vi "S4GUI_003.vi"(7 "Tab ObsEng":enum32{"Obs", "CCD modes", "Guider", "Eng"}(tab)) -> ()   [LabVIEW 2018] (continued)
            n4197 = call "Write WPROT.vi"("error in (no error)"=w9692, "Opt_Selector.lvclass"=w9693, "Instrument in"=w9713) -> ("error out"=w9709:errorcluster, "Instrument out"=w9708:refnum<class "Instrument.lvclass">)  [unwired: 7 in]
            n4198 = call "Write Instrument.lvclass.vi"("error in (no error)"=w9709, "Instrument.lvclass"=w9708, "S4ACS_GUI in"=w9715) -> ("error out"=w9703:errorcluster, "S4ACS_GUI out"=w9691:refnum<class "S4GUI.lvclass">)  [unwired: 7 in]
          }
          frame Enabled {
            w9742 = FALSE ("Wait Until Done")
            n4199 = call <vilib>:"Application Directory.vi"() -> ("Application Directory"=w9737:path)
            n4200 = Build Path(base path=w9737, name or relative path="MsgAbort2.vi") -> (appended path=w9745:path)
            n4201 = Open VI Reference(vi path=w9745, error in (no error)=w9740) -> (vi reference=w9744:refnum<vi>, error out=w9743:errorcluster)  [unwired: 4 in]
            n4202 = invoke class="VI" method="Run VI"(reference=w9744, error in=w9743, "Wait until done"=w9742, "Auto Dispose Ref"=w9742) -> (error out=w9738:errorcluster)  [unwired: 1 in, 4 out]
          }
        }
      }
      event "Abort ch3": Value Change {
        n4203 = event-data() -> ()  [unwired: 1 in, 6 out]
        n4204 = disable-structure shown="Enabled" {
          disable-tunnel: w9749 -> [w9782 w9798]
          disable-tunnel: w9748 -> [w9780 w9799]
          disable-tunnel: [w9762 w9797] -> w9747
          disable-tunnel: [w9750 w9798] -> w9746
          frame Disabled {
            # "Para movimento \nda lamina retardadora"
            # "Restaura a última sequência de lâminas"
            n4205 = call-dynamic "Read AcquisitionC.vi"("error in (no error)"=w9780, "S4ACS_GUI in"=w9782) -> ("error out"=w9785:errorcluster, "Acquisition.lvclass"=w9784:refnum<class "Acquisition.lvclass">, "S4ACS_GUI out"=w9781:refnum<class "S4GUI.lvclass">)  [unwired: 7 in]
            n4206 = call-dynamic "Read Channel.vi"("error in (no error)"=w9785, "Acquisition in"=w9784) -> ("error out"=w9787:errorcluster, "Channel.lvclass"=w9786:refnum<class "Channel.lvclass">, "Acquisition out"=w9793:refnum<class "Acquisition.lvclass">)  [unwired: 7 in]
            n4207 = call-dynamic "Read State Machine.vi"("error in (no error)"=w9787, "Device in"=w9786) -> ("error out"=w9789:errorcluster, "State Machine.lvclass"=w9788:refnum<class "State Machine.lvclass">, "Device out"=w9791:refnum<class "Channel.lvclass">)  [unwired: 7 in]
            n4208 = call "Next State.vi"("error in (no error)"=w9789, "New_State"=u32 80, "State Machine in"=w9788) -> ("error out"=w9792:errorcluster, "State Machine out"=w9790:refnum<class "State Machine.lvclass">)  [unwired: 7 in]
            n4209 = call-dynamic "Write State Machine.vi"("error in (no error)"=w9792, "State Machine.lvclass"=w9790, "Device in"=w9791) -> ("error out"=w9794:errorcluster, "Device out"=w9795:refnum<class "Channel.lvclass">)  [unwired: 7 in]
            n4210 = call-dynamic "Write Channel.vi"("error in (no error)"=w9794, "Channel.lvclass"=w9795, "Acquisition in"=w9793) -> ("error out"=w9777:errorcluster, "Acquisition out"=w9778:refnum<class "Acquisition.lvclass">)  [unwired: 7 in]
            n4211 = call-dynamic "Write Acq_state.vi"("error in (no error)"=w9777, "Acq_state"=u32 0, "Acquisition in"=w9778) -> ("error out"=w9776:errorcluster, "Acquisition out"=w9775:refnum<class "Acquisition.lvclass">)  [unwired: 7 in]
            n4212 = call-dynamic "Write AcquisitionC.vi"("error in (no error)"=w9776, "Acquisition.lvclass"=w9775, "S4ACS_GUI in"=w9781) -> ("error out"=w9763:errorcluster, "S4ACS_GUI out"=w9761:refnum<class "S4GUI.lvclass">)  [unwired: 7 in]
            n4213 = call "Read Instrument.lvclass.vi"("error in (no error)"=w9763, "S4ACS_GUI in"=w9761) -> ("error out"=w9770:errorcluster, "Instrument.lvclass"=w9773:refnum<class "Instrument.lvclass">, "S4ACS_GUI out"=w9774:refnum<class "S4GUI.lvclass">)  [unwired: 7 in]
            n4214 = call "Read WPROT.vi"("error in (no error)"=w9770, "Instrument in"=w9773) -> ("error out"=w9769:errorcluster, "Opt_Selector.lvclass"=w9771:refnum<class "Opt_Selector.lvclass">, "Instrument out"=w9772:refnum<class "Instrument.lvclass">)  [unwired: 7 in]
            n4215 = call-dynamic "Read sequencia_ant.vi"("error in (no error)"=w9769, "Opt_Selector in"=w9771) -> ("error out"=w9765:errorcluster, "sequencia_ant"=w9764:u16, "Opt_Selector out"=w9766:refnum<class "Opt_Selector.lvclass">)  [unwired: 7 in]
            n4216 = call-dynamic "Write sequencia.vi"("error in (no error)"=w9765, "sequencia"=w9764, "Opt_Selector in"=w9766) -> ("error out"=w9754:errorcluster, "Opt_Selector out"=w9755:refnum<class "Opt_Selector.lvclass">)  [unwired: 7 in]
            n4217 = call-dynamic "Read State Machine.vi"("error in (no error)"=w9754, "Device in"=w9755) -> ("error out"=w9757:errorcluster, "State Machine.lvclass"=w9760:refnum<class "State Machine.lvclass">, "Device out"=w9753:refnum<class "Opt_Selector.lvclass">)  [unwired: 7 in]
            n4218 = call "Next State.vi"("error in (no error)"=w9757, "New_State"=10, "State Machine in"=w9760) -> ("error out"=w9756:errorcluster, "State Machine out"=w9759:refnum<class "State Machine.lvclass">)  [unwired: 7 in]
            n4219 = call-dynamic "Write State Machine.vi"("error in (no error)"=w9756, "State Machine.lvclass"=w9759, "Device in"=w9753) -> ("error out"=w9751:errorcluster, "Device out"=w9752:refnum<class "Opt_Selector.lvclass">)  [unwired: 7 in]
            n4220 = call "Write WPROT.vi"("error in (no error)"=w9751, "Opt_Selector.lvclass"=w9752, "Instrument in"=w9772) -> ("error out"=w9768:errorcluster, "Instrument out"=w9767:refnum<class "Instrument.lvclass">)  [unwired: 7 in]
            n4221 = call "Write Instrument.lvclass.vi"("error in (no error)"=w9768, "Instrument.lvclass"=w9767, "S4ACS_GUI in"=w9774) -> ("error out"=w9762:errorcluster, "S4ACS_GUI out"=w9750:refnum<class "S4GUI.lvclass">)  [unwired: 7 in]
          }
          frame Enabled {
            w9801 = FALSE ("Wait Until Done")
            n4222 = call <vilib>:"Application Directory.vi"() -> ("Application Directory"=w9796:path)
            n4223 = Build Path(base path=w9796, name or relative path="MsgAbort3.vi") -> (appended path=w9804:path)
            n4224 = Open VI Reference(vi path=w9804, error in (no error)=w9799) -> (vi reference=w9803:refnum<vi>, error out=w9802:errorcluster)  [unwired: 4 in]
            n4225 = invoke class="VI" method="Run VI"(reference=w9803, error in=w9802, "Wait until done"=w9801, "Auto Dispose Ref"=w9801) -> (error out=w9797:errorcluster)  [unwired: 1 in, 4 out]
          }
        }
      }
      event "Abort ch4": Value Change {
        n4226 = event-data() -> ()  [unwired: 1 in, 6 out]
        n4227 = disable-structure shown="Enabled" {
          disable-tunnel: w9808 -> [w9841 w9857]
          disable-tunnel: w9807 -> [w9839 w9858]
          disable-tunnel: [w9821 w9856] -> w9806
          disable-tunnel: [w9809 w9857] -> w9805
          frame Disabled {
            # "Para movimento \nda lamina retardadora"
            # "Restaura a última sequência de lâminas"
            n4228 = call-dynamic "Read AcquisitionD.vi"("error in (no error)"=w9839, "S4ACS_GUI in"=w9841) -> ("error out"=w9844:errorcluster, "Acquisition.lvclass"=w9843:refnum<class "Acquisition.lvclass">, "S4ACS_GUI out"=w9840:refnum<class "S4GUI.lvclass">)  [unwired: 7 in]
            n4229 = call-dynamic "Read Channel.vi"("error in (no error)"=w9844, "Acquisition in"=w9843) -> ("error out"=w9846:errorcluster, "Channel.lvclass"=w9845:refnum<class "Channel.lvclass">, "Acquisition out"=w9852:refnum<class "Acquisition.lvclass">)  [unwired: 7 in]
            n4230 = call-dynamic "Read State Machine.vi"("error in (no error)"=w9846, "Device in"=w9845) -> ("error out"=w9848:errorcluster, "State Machine.lvclass"=w9847:refnum<class "State Machine.lvclass">, "Device out"=w9850:refnum<class "Channel.lvclass">)  [unwired: 7 in]
            n4231 = call "Next State.vi"("error in (no error)"=w9848, "New_State"=u32 80, "State Machine in"=w9847) -> ("error out"=w9851:errorcluster, "State Machine out"=w9849:refnum<class "State Machine.lvclass">)  [unwired: 7 in]
            n4232 = call-dynamic "Write State Machine.vi"("error in (no error)"=w9851, "State Machine.lvclass"=w9849, "Device in"=w9850) -> ("error out"=w9853:errorcluster, "Device out"=w9854:refnum<class "Channel.lvclass">)  [unwired: 7 in]
            n4233 = call-dynamic "Write Channel.vi"("error in (no error)"=w9853, "Channel.lvclass"=w9854, "Acquisition in"=w9852) -> ("error out"=w9836:errorcluster, "Acquisition out"=w9837:refnum<class "Acquisition.lvclass">)  [unwired: 7 in]
            n4234 = call-dynamic "Write Acq_state.vi"("error in (no error)"=w9836, "Acq_state"=u32 0, "Acquisition in"=w9837) -> ("error out"=w9835:errorcluster, "Acquisition out"=w9834:refnum<class "Acquisition.lvclass">)  [unwired: 7 in]
            n4235 = call-dynamic "Write AcquisitionD.vi"("error in (no error)"=w9835, "Acquisition.lvclass"=w9834, "S4ACS_GUI in"=w9840) -> ("error out"=w9822:errorcluster, "S4ACS_GUI out"=w9820:refnum<class "S4GUI.lvclass">)  [unwired: 7 in]
            n4236 = call "Read Instrument.lvclass.vi"("error in (no error)"=w9822, "S4ACS_GUI in"=w9820) -> ("error out"=w9829:errorcluster, "Instrument.lvclass"=w9832:refnum<class "Instrument.lvclass">, "S4ACS_GUI out"=w9833:refnum<class "S4GUI.lvclass">)  [unwired: 7 in]
            n4237 = call "Read WPROT.vi"("error in (no error)"=w9829, "Instrument in"=w9832) -> ("error out"=w9828:errorcluster, "Opt_Selector.lvclass"=w9830:refnum<class "Opt_Selector.lvclass">, "Instrument out"=w9831:refnum<class "Instrument.lvclass">)  [unwired: 7 in]
            n4238 = call-dynamic "Read sequencia_ant.vi"("error in (no error)"=w9828, "Opt_Selector in"=w9830) -> ("error out"=w9824:errorcluster, "sequencia_ant"=w9823:u16, "Opt_Selector out"=w9825:refnum<class "Opt_Selector.lvclass">)  [unwired: 7 in]
            n4239 = call-dynamic "Write sequencia.vi"("error in (no error)"=w9824, "sequencia"=w9823, "Opt_Selector in"=w9825) -> ("error out"=w9813:errorcluster, "Opt_Selector out"=w9814:refnum<class "Opt_Selector.lvclass">)  [unwired: 7 in]
            n4240 = call-dynamic "Read State Machine.vi"("error in (no error)"=w9813, "Device in"=w9814) -> ("error out"=w9816:errorcluster, "State Machine.lvclass"=w9819:refnum<class "State Machine.lvclass">, "Device out"=w9812:refnum<class "Opt_Selector.lvclass">)  [unwired: 7 in]
            n4241 = call "Next State.vi"("error in (no error)"=w9816, "New_State"=10, "State Machine in"=w9819) -> ("error out"=w9815:errorcluster, "State Machine out"=w9818:refnum<class "State Machine.lvclass">)  [unwired: 7 in]
            n4242 = call-dynamic "Write State Machine.vi"("error in (no error)"=w9815, "State Machine.lvclass"=w9818, "Device in"=w9812) -> ("error out"=w9810:errorcluster, "Device out"=w9811:refnum<class "Opt_Selector.lvclass">)  [unwired: 7 in]
            n4243 = call "Write WPROT.vi"("error in (no error)"=w9810, "Opt_Selector.lvclass"=w9811, "Instrument in"=w9831) -> ("error out"=w9827:errorcluster, "Instrument out"=w9826:refnum<class "Instrument.lvclass">)  [unwired: 7 in]
            n4244 = call "Write Instrument.lvclass.vi"("error in (no error)"=w9827, "Instrument.lvclass"=w9826, "S4ACS_GUI in"=w9833) -> ("error out"=w9821:errorcluster, "S4ACS_GUI out"=w9809:refnum<class "S4GUI.lvclass">)  [unwired: 7 in]
          }
          frame Enabled {
            w9860 = FALSE ("Wait Until Done")
            n4245 = call <vilib>:"Application Directory.vi"() -> ("Application Directory"=w9855:path)
            n4246 = Build Path(base path=w9855, name or relative path="MsgAbort4.vi") -> (appended path=w9863:path)
            n4247 = Open VI Reference(vi path=w9863, error in (no error)=w9858) -> (vi reference=w9862:refnum<vi>, error out=w9861:errorcluster)  [unwired: 4 in]
            n4248 = invoke class="VI" method="Run VI"(reference=w9862, error in=w9861, "Wait until done"=w9860, "Auto Dispose Ref"=w9860) -> (error out=w9856:errorcluster)  [unwired: 1 in, 4 out]
          }
        }
      }
      event "SyncBox": Value Change {
        n4249 = event-data() -> ()  [unwired: 1 in, 4 out]
        n4250 = call-dynamic "Read Sync Box.lvclass.vi"("error in (no error)"=w9866, "SPARC4_AC in"=w9867) -> ("error out"=w9882:errorcluster, "Sync Box.lvclass"=w9883:refnum<class "Sync Box.lvclass">, "SPARC4_AC out"=w9871:refnum<class "S4GUI.lvclass">)  [unwired: 7 in]
        n4251 = call-dynamic "Read Trigger.lvclass.vi"("error in (no error)"=w9882, "Sync Box in"=w9883) -> ("error out"=w9880:errorcluster, "Trigger.lvclass"=w9881:refnum<class "Trigger.lvclass">, "Sync Box out"=w9874:refnum<class "Sync Box.lvclass">)  [unwired: 7 in]
        n4252 = call-dynamic "Read State Machine.vi"("error in (no error)"=w9880, "Device in"=w9881) -> ("error out"=w9878:errorcluster, "State Machine.lvclass"=w9879:refnum<class "State Machine.lvclass">, "Device out"=w9875:refnum<class "Trigger.lvclass">)  [unwired: 7 in]
        n4253 = call "Next State.vi"("error in (no error)"=w9878, "New_State"=u32 1, "State Machine in"=w9879) -> ("error out"=w9873:errorcluster, "State Machine out"=w9876:refnum<class "State Machine.lvclass">)  [unwired: 7 in]
        n4254 = call-dynamic "Write State Machine.vi"("error in (no error)"=w9873, "State Machine.lvclass"=w9876, "Device in"=w9875) -> ("error out"=w9869:errorcluster, "Device out"=w9868:refnum<class "Trigger.lvclass">)  [unwired: 7 in]
        n4255 = call-dynamic "Write Trigger.lvclass.vi"("error in (no error)"=w9869, "Trigger.lvclass"=w9868, "Sync Box in"=w9874) -> ("error out"=w9870:errorcluster, "Sync Box out"=w9872:refnum<class "Sync Box.lvclass">)  [unwired: 7 in]
        n4256 = call-dynamic "Write Sync Box.lvclass.vi"("error in (no error)"=w9870, "Sync Box.lvclass"=w9872, "SPARC4_AC in"=w9871) -> ("error out"=w9865:errorcluster, "SPARC4_AC out"=w9864:refnum<class "S4GUI.lvclass">)  [unwired: 7 in]
      }
      event "Fire manual", "Fire": Value Change {
        n4257 = event-data() -> ()  [unwired: 1 in, 4 out]
        n4258 = call-dynamic "Read Sync Box.lvclass.vi"("error in (no error)"=w9886, "SPARC4_AC in"=w9887) -> ("error out"=w9902:errorcluster, "Sync Box.lvclass"=w9903:refnum<class "Sync Box.lvclass">, "SPARC4_AC out"=w9891:refnum<class "S4GUI.lvclass">)  [unwired: 7 in]
        n4259 = call-dynamic "Read Trigger.lvclass.vi"("error in (no error)"=w9902, "Sync Box in"=w9903) -> ("error out"=w9900:errorcluster, "Trigger.lvclass"=w9901:refnum<class "Trigger.lvclass">, "Sync Box out"=w9894:refnum<class "Sync Box.lvclass">)  [unwired: 7 in]
        n4260 = call-dynamic "Read State Machine.vi"("error in (no error)"=w9900, "Device in"=w9901) -> ("error out"=w9898:errorcluster, "State Machine.lvclass"=w9899:refnum<class "State Machine.lvclass">, "Device out"=w9895:refnum<class "Trigger.lvclass">)  [unwired: 7 in]
        n4261 = call "Next State.vi"("error in (no error)"=w9898, "New_State"=u32 40, "State Machine in"=w9899) -> ("error out"=w9893:errorcluster, "State Machine out"=w9896:refnum<class "State Machine.lvclass">)  [unwired: 7 in]
        n4262 = call-dynamic "Write State Machine.vi"("error in (no error)"=w9893, "State Machine.lvclass"=w9896, "Device in"=w9895) -> ("error out"=w9889:errorcluster, "Device out"=w9888:refnum<class "Trigger.lvclass">)  [unwired: 7 in]
        n4263 = call-dynamic "Write Trigger.lvclass.vi"("error in (no error)"=w9889, "Trigger.lvclass"=w9888, "Sync Box in"=w9894) -> ("error out"=w9890:errorcluster, "Sync Box out"=w9892:refnum<class "Sync Box.lvclass">)  [unwired: 7 in]
        n4264 = call-dynamic "Write Sync Box.lvclass.vi"("error in (no error)"=w9890, "Sync Box.lvclass"=w9892, "SPARC4_AC in"=w9891) -> ("error out"=w9885:errorcluster, "SPARC4_AC out"=w9884:refnum<class "S4GUI.lvclass">)  [unwired: 7 in]
      }
      event "Select Trigger Mode": Value Change {
        n4265 = event-data() -> ("NewVal"=w9905:bool)  [unwired: 1 in, 2 out]
        n4266 = call-dynamic "Read Sync Box.lvclass.vi"("error in (no error)"=w9913, "SPARC4_AC in"=w9914) -> ("error out"=w9925:errorcluster, "Sync Box.lvclass"=w9926:refnum<class "Sync Box.lvclass">, "SPARC4_AC out"=w9918:refnum<class "S4GUI.lvclass">)  [unwired: 7 in]
        n4267 = call-dynamic "Read Trigger.lvclass.vi"("error in (no error)"=w9925, "Sync Box in"=w9926) -> ("error out"=w9906:errorcluster, "Trigger.lvclass"=w9909:refnum<class "Trigger.lvclass">, "Sync Box out"=w9921:refnum<class "Sync Box.lvclass">)  [unwired: 7 in]
        n4268 = call-dynamic "Write Trigger Mode Target.vi"("error in (no error)"=w9906, "Trigger Mode Target"=w9905, "Trigger in"=w9909) -> ("error out"=w9907:errorcluster, "Trigger out"=w9908:refnum<class "Trigger.lvclass">)  [unwired: 7 in]
        n4269 = call-dynamic "Read State Machine.vi"("error in (no error)"=w9907, "Device in"=w9908) -> ("error out"=w9910:errorcluster, "State Machine.lvclass"=w9911:refnum<class "State Machine.lvclass">, "Device out"=w9922:refnum<class "Trigger.lvclass">)  [unwired: 7 in]
        n4270 = call "Next State.vi"("error in (no error)"=w9910, "New_State"=u32 30, "State Machine in"=w9911) -> ("error out"=w9920:errorcluster, "State Machine out"=w9923:refnum<class "State Machine.lvclass">)  [unwired: 7 in]
        n4271 = call-dynamic "Write State Machine.vi"("error in (no error)"=w9920, "State Machine.lvclass"=w9923, "Device in"=w9922) -> ("error out"=w9916:errorcluster, "Device out"=w9915:refnum<class "Trigger.lvclass">)  [unwired: 7 in]
        n4272 = call-dynamic "Write Trigger.lvclass.vi"("error in (no error)"=w9916, "Trigger.lvclass"=w9915, "Sync Box in"=w9921) -> ("error out"=w9917:errorcluster, "Sync Box out"=w9919:refnum<class "Sync Box.lvclass">)  [unwired: 7 in]
        n4273 = call-dynamic "Write Sync Box.lvclass.vi"("error in (no error)"=w9917, "Sync Box.lvclass"=w9919, "SPARC4_AC in"=w9918) -> ("error out"=w9912:errorcluster, "SPARC4_AC out"=w9904:refnum<class "S4GUI.lvclass">)  [unwired: 7 in]
      }
      event "Set SyncBox": Value Change {
        n4274 = event-data() -> ()  [unwired: 1 in, 4 out]
        n4275 = call-dynamic "Read Sync Box.lvclass.vi"("error in (no error)"=w9929, "SPARC4_AC in"=w9930) -> ("error out"=w9945:errorcluster, "Sync Box.lvclass"=w9946:refnum<class "Sync Box.lvclass">, "SPARC4_AC out"=w9934:refnum<class "S4GUI.lvclass">)  [unwired: 7 in]
        n4276 = call-dynamic "Read Trigger.lvclass.vi"("error in (no error)"=w9945, "Sync Box in"=w9946) -> ("error out"=w9943:errorcluster, "Trigger.lvclass"=w9944:refnum<class "Trigger.lvclass">, "Sync Box out"=w9937:refnum<class "Sync Box.lvclass">)  [unwired: 7 in]
        n4277 = call-dynamic "Read State Machine.vi"("error in (no error)"=w9943, "Device in"=w9944) -> ("error out"=w9941:errorcluster, "State Machine.lvclass"=w9942:refnum<class "State Machine.lvclass">, "Device out"=w9938:refnum<class "Trigger.lvclass">)  [unwired: 7 in]
        n4278 = call "Next State.vi"("error in (no error)"=w9941, "New_State"=u32 10, "State Machine in"=w9942) -> ("error out"=w9936:errorcluster, "State Machine out"=w9939:refnum<class "State Machine.lvclass">)  [unwired: 7 in]
        n4279 = call-dynamic "Write State Machine.vi"("error in (no error)"=w9936, "State Machine.lvclass"=w9939, "Device in"=w9938) -> ("error out"=w9932:errorcluster, "Device out"=w9931:refnum<class "Trigger.lvclass">)  [unwired: 7 in]
        n4280 = call-dynamic "Write Trigger.lvclass.vi"("error in (no error)"=w9932, "Trigger.lvclass"=w9931, "Sync Box in"=w9937) -> ("error out"=w9933:errorcluster, "Sync Box out"=w9935:refnum<class "Sync Box.lvclass">)  [unwired: 7 in]
        n4281 = call-dynamic "Write Sync Box.lvclass.vi"("error in (no error)"=w9933, "Sync Box.lvclass"=w9935, "SPARC4_AC in"=w9934) -> ("error out"=w9928:errorcluster, "SPARC4_AC out"=w9927:refnum<class "S4GUI.lvclass">)  [unwired: 7 in]
      }
      event "Set Focus": Value Change {
        n4282 = event-data() -> ("NewVal"=w9947:bool)  [unwired: 1 in]
        n4283 = case shown="True" w9947 {
          tunnel: w9951 -> [w9953 w9962]
          tunnel: w9950 -> [w9952 w9961]
          tunnel: [w9952 w9960] -> w9949
          tunnel: [w9953 w9959] -> w9948
          frame False {
          }
          frame True {
            n4284 = call-dynamic "Read TelFocus.lvclass.vi"("error in (no error)"=w9961, "S4GUI in"=w9962) -> ("error out"=w9975:errorcluster, "TelFocus.lvclass"=w9976:refnum<class "TelFocus.lvclass">, "S4GUI out"=w9966:refnum<class "S4GUI.lvclass">)  [unwired: 7 in]
            n4285 = call-dynamic "Read SecMirror.lvclass.vi"("error in (no error)"=w9975, "TelFocus in"=w9976) -> ("error out"=w9955:errorcluster, "SecMirror.lvclass"=w9958:refnum<class "SecMirror.lvclass">, "TelFocus out"=w9969:refnum<class "TelFocus.lvclass">)  [unwired: 7 in]
            n4286 = call-dynamic "Write target.vi"("error in (no error)"=w9955, "target"="Target focus", "SecMirror in"=w9958) -> ("error out"=w9954:errorcluster, "SecMirror out"=w9957:refnum<class "SecMirror.lvclass">)  [unwired: 7 in]
            n4287 = call-dynamic "Read State Machine.vi"("error in (no error)"=w9954, "Device in"=w9957) -> ("error out"=w9973:errorcluster, "State Machine.lvclass"=w9974:refnum<class "State Machine.lvclass">, "Device out"=w9970:refnum<class "SecMirror.lvclass">)  [unwired: 7 in]
            n4288 = call "Next State.vi"("error in (no error)"=w9973, "New_State"=1, "State Machine in"=w9974) -> ("error out"=w9968:errorcluster, "State Machine out"=w9971:refnum<class "State Machine.lvclass">)  [unwired: 7 in]
            n4289 = call-dynamic "Write State Machine.vi"("error in (no error)"=w9968, "State Machine.lvclass"=w9971, "Device in"=w9970) -> ("error out"=w9964:errorcluster, "Device out"=w9963:refnum<class "SecMirror.lvclass">)  [unwired: 7 in]
            n4290 = call-dynamic "Write SecMirror.lvclass.vi"("error in (no error)"=w9964, "SecMirror.lvclass"=w9963, "TelFocus in"=w9969) -> ("error out"=w9965:errorcluster, "TelFocus out"=w9967:refnum<class "TelFocus.lvclass">)  [unwired: 7 in]
            n4291 = call-dynamic "Write TelFocus.lvclass.vi"("error in (no error)"=w9965, "TelFocus.lvclass"=w9967, "S4GUI in"=w9966) -> ("error out"=w9960:errorcluster, "S4GUI out"=w9959:refnum<class "S4GUI.lvclass">)  [unwired: 7 in]
          }
        }
      }
      event "Set Focus 2": Value Change {
        n4292 = event-data() -> ("NewVal"=w9977:bool)  [unwired: 1 in]
        n4293 = case shown="True" w9977 {
          tunnel: w9981 -> [w9983 w9992]
          tunnel: w9980 -> [w9982 w9991]
          tunnel: [w9982 w9990] -> w9979
          tunnel: [w9983 w9989] -> w9978
          frame False {
          }
          frame True {
            n4294 = call-dynamic "Read TelFocus.lvclass.vi"("error in (no error)"=w9991, "S4GUI in"=w9992) -> ("error out"=w10005:errorcluster, "TelFocus.lvclass"=w10006:refnum<class "TelFocus.lvclass">, "S4GUI out"=w9996:refnum<class "S4GUI.lvclass">)  [unwired: 7 in]
            n4295 = call-dynamic "Read SecMirror.lvclass.vi"("error in (no error)"=w10005, "TelFocus in"=w10006) -> ("error out"=w9986:errorcluster, "SecMirror.lvclass"=w9988:refnum<class "SecMirror.lvclass">, "TelFocus out"=w9999:refnum<class "TelFocus.lvclass">)  [unwired: 7 in]
            n4296 = call-dynamic "Write target.vi"("error in (no error)"=w9986, "target"="Target focus 2", "SecMirror in"=w9988) -> ("error out"=w9985:errorcluster, "SecMirror out"=w9987:refnum<class "SecMirror.lvclass">)  [unwired: 7 in]
            n4297 = call-dynamic "Read State Machine.vi"("error in (no error)"=w9985, "Device in"=w9987) -> ("error out"=w10003:errorcluster, "State Machine.lvclass"=w10004:refnum<class "State Machine.lvclass">, "Device out"=w10000:refnum<class "SecMirror.lvclass">)  [unwired: 7 in]
            n4298 = call "Next State.vi"("error in (no error)"=w10003, "New_State"=1, "State Machine in"=w10004) -> ("error out"=w9998:errorcluster, "State Machine out"=w10001:refnum<class "State Machine.lvclass">)  [unwired: 7 in]
            n4299 = call-dynamic "Write State Machine.vi"("error in (no error)"=w9998, "State Machine.lvclass"=w10001, "Device in"=w10000) -> ("error out"=w9994:errorcluster, "Device out"=w9993:refnum<class "SecMirror.lvclass">)  [unwired: 7 in]
            n4300 = call-dynamic "Write SecMirror.lvclass.vi"("error in (no error)"=w9994, "SecMirror.lvclass"=w9993, "TelFocus in"=w9999) -> ("error out"=w9995:errorcluster, "TelFocus out"=w9997:refnum<class "TelFocus.lvclass">)  [unwired: 7 in]
            n4301 = call-dynamic "Write TelFocus.lvclass.vi"("error in (no error)"=w9995, "TelFocus.lvclass"=w9997, "S4GUI in"=w9996) -> ("error out"=w9990:errorcluster, "S4GUI out"=w9989:refnum<class "S4GUI.lvclass">)  [unwired: 7 in]
          }
        }
      }
      event "Stop Focus", "Stop Focus 2": Value Change {
        n4302 = event-data() -> ("NewVal"=w10007:bool)  [unwired: 1 in]
        n4303 = case shown="True" w10007 {
          tunnel: w10011 -> [w10013 w10019]
          tunnel: w10010 -> [w10012 w10018]
          tunnel: [w10012 w10017] -> w10009
          tunnel: [w10013 w10016] -> w10008
          frame False {
          }
          frame True {
            n4304 = call-dynamic "Read TelFocus.lvclass.vi"("error in (no error)"=w10018, "S4GUI in"=w10019) -> ("error out"=w10032:errorcluster, "TelFocus.lvclass"=w10033:refnum<class "TelFocus.lvclass">, "S4GUI out"=w10023:refnum<class "S4GUI.lvclass">)  [unwired: 7 in]
            n4305 = call-dynamic "Read SecMirror.lvclass.vi"("error in (no error)"=w10032, "TelFocus in"=w10033) -> ("error out"=w10014:errorcluster, "SecMirror.lvclass"=w10015:refnum<class "SecMirror.lvclass">, "TelFocus out"=w10026:refnum<class "TelFocus.lvclass">)  [unwired: 7 in]
            n4306 = call-dynamic "Read State Machine.vi"("error in (no error)"=w10014, "Device in"=w10015) -> ("error out"=w10030:errorcluster, "State Machine.lvclass"=w10031:refnum<class "State Machine.lvclass">, "Device out"=w10027:refnum<class "SecMirror.lvclass">)  [unwired: 7 in]
            n4307 = call "Next State.vi"("error in (no error)"=w10030, "New_State"=10, "State Machine in"=w10031) -> ("error out"=w10025:errorcluster, "State Machine out"=w10028:refnum<class "State Machine.lvclass">)  [unwired: 7 in]
            n4308 = call-dynamic "Write State Machine.vi"("error in (no error)"=w10025, "State Machine.lvclass"=w10028, "Device in"=w10027) -> ("error out"=w10021:errorcluster, "Device out"=w10020:refnum<class "SecMirror.lvclass">)  [unwired: 7 in]
            n4309 = call-dynamic "Write SecMirror.lvclass.vi"("error in (no error)"=w10021, "SecMirror.lvclass"=w10020, "TelFocus in"=w10026) -> ("error out"=w10022:errorcluster, "TelFocus out"=w10024:refnum<class "TelFocus.lvclass">)  [unwired: 7 in]
            n4310 = call-dynamic "Write TelFocus.lvclass.vi"("error in (no error)"=w10022, "TelFocus.lvclass"=w10024, "S4GUI in"=w10023) -> ("error out"=w10017:errorcluster, "S4GUI out"=w10016:refnum<class "S4GUI.lvclass">)  [unwired: 7 in]
          }
        }
      }
      event "cooler ON 1": Value Change {
        n4311 = event-data() -> ("NewVal"=w10034:bool)  [unwired: 1 in]
        n4312 = case shown="True" w10034 {
          tunnel: [w10039 w10074] -> w10038
          tunnel: [w10040 w10073] -> w10037
          tunnel: w10036 -> [w10040 w10044]
          tunnel: w10035 -> [w10039 w10043]
          frame False {
          }
          frame True {
            w10042 = i16 1 items=["Cooler OFF", "Cooler ON"] ("Cooler ON/OFF")
            n4313 = Concatenate Strings("SET COOLER " ("User Event"), "ON ", "CLICKED - CH1" ("User Event")) -> (w10046:string)
            n4314 = call-dynamic "Write User Event.vi"("error in (no error)"=w10043, "User Event"=w10046, "S4GUI in"=w10044) -> ("error out"=w10047:errorcluster, "S4GUI out"=w10049:refnum<class "S4GUI.lvclass">)  [unwired: 7 in]
            n4315 = call-dynamic "Read AcquisitionA.vi"("error in (no error)"=w10047, "S4ACS_GUI in"=w10049) -> ("error out"=w10071:errorcluster, "Acquisition.lvclass"=w10072:refnum<class "Acquisition.lvclass">, "S4ACS_GUI out"=w10062:refnum<class "S4GUI.lvclass">)  [unwired: 7 in]
            n4316 = call-dynamic "Read Channel.vi"("error in (no error)"=w10071, "Acquisition in"=w10072) -> ("error out"=w10055:errorcluster, "Channel.lvclass"=w10059:refnum<class "Channel.lvclass">, "Acquisition out"=w10065:refnum<class "Acquisition.lvclass">)  [unwired: 7 in]
            n4317 = call-dynamic "Read Interface.vi"("error in (no error)"=w10055, "Channel in"=w10059) -> ("error out"=w10050:errorcluster, "Interface.lvclass"=w10051:refnum<class "Interface.lvclass">, "Channel out"=w10058:refnum<class "Channel.lvclass">)  [unwired: 7 in]
            n4318 = call-dynamic "Write Cooler ON_OFF.vi"("error in (no error)"=w10050, "Cooler ON/OFF"=w10042, "Interface in"=w10051) -> ("error out"=w10054:errorcluster, "Interface out"=w10056:refnum<class "Interface.lvclass">)  [unwired: 7 in]
            n4319 = call-dynamic "Write Interface.vi"("error in (no error)"=w10054, "Interface.lvclass"=w10056, "Channel in"=w10058) -> ("error out"=w10053:errorcluster, "Channel out"=w10057:refnum<class "Channel.lvclass">)  [unwired: 7 in]
            n4320 = call-dynamic "Read State Machine.vi"("error in (no error)"=w10053, "Device in"=w10057) -> ("error out"=w10069:errorcluster, "State Machine.lvclass"=w10070:refnum<class "State Machine.lvclass">, "Device out"=w10066:refnum<class "Channel.lvclass">)  [unwired: 7 in]
            n4321 = call "Next State.vi"("error in (no error)"=w10069, "New_State"=u32 30, "State Machine in"=w10070) -> ("error out"=w10064:errorcluster, "State Machine out"=w10067:refnum<class "State Machine.lvclass">)  [unwired: 7 in]
            n4322 = call-dynamic "Write State Machine.vi"("error in (no error)"=w10064, "State Machine.lvclass"=w10067, "Device in"=w10066) -> ("error out"=w10060:errorcluster, "Device out"=w10052:refnum<class "Channel.lvclass">)  [unwired: 7 in]
            n4323 = call-dynamic "Write Channel.vi"("error in (no error)"=w10060, "Channel.lvclass"=w10052, "Acquisition in"=w10065) -> ("error out"=w10061:errorcluster, "Acquisition out"=w10063:refnum<class "Acquisition.lvclass">)  [unwired: 7 in]
            n4324 = call-dynamic "Write AcquisitionA.vi"("error in (no error)"=w10061, "Acquisition.lvclass"=w10063, "S4ACS_GUI in"=w10062) -> ("error out"=w10074:errorcluster, "S4ACS_GUI out"=w10073:refnum<class "S4GUI.lvclass">)  [unwired: 7 in]
          }
        }
      }
      event "cooler ON 2": Value Change {
        n4325 = event-data() -> ("NewVal"=w10075:bool)  [unwired: 1 in]
        n4326 = case shown="True" w10075 {
          tunnel: [w10080 w10115] -> w10079
          tunnel: [w10081 w10114] -> w10078
          tunnel: w10077 -> [w10081 w10085]
          tunnel: w10076 -> [w10080 w10084]
          frame False {
          }
          frame True {
            w10083 = i16 1 items=["Cooler OFF", "Cooler ON"] ("Cooler ON/OFF")
            n4327 = Concatenate Strings("SET COOLER " ("User Event"), "ON ", "CLICKED - CH2" ("User Event")) -> (w10087:string)
            n4328 = call-dynamic "Write User Event.vi"("error in (no error)"=w10084, "User Event"=w10087, "S4GUI in"=w10085) -> ("error out"=w10088:errorcluster, "S4GUI out"=w10090:refnum<class "S4GUI.lvclass">)  [unwired: 7 in]
            n4329 = call "Read AcquisitionB.vi"("error in (no error)"=w10088, "S4ACS_GUI in"=w10090) -> ("error out"=w10112:errorcluster, "Acquisition.lvclass"=w10113:refnum<class "Acquisition.lvclass">, "S4ACS_GUI out"=w10103:refnum<class "S4GUI.lvclass">)  [unwired: 7 in]
            n4330 = call-dynamic "Read Channel.vi"("error in (no error)"=w10112, "Acquisition in"=w10113) -> ("error out"=w10096:errorcluster, "Channel.lvclass"=w10100:refnum<class "Channel.lvclass">, "Acquisition out"=w10106:refnum<class "Acquisition.lvclass">)  [unwired: 7 in]
            n4331 = call-dynamic "Read Interface.vi"("error in (no error)"=w10096, "Channel in"=w10100) -> ("error out"=w10091:errorcluster, "Interface.lvclass"=w10092:refnum<class "Interface.lvclass">, "Channel out"=w10099:refnum<class "Channel.lvclass">)  [unwired: 7 in]
            n4332 = call-dynamic "Write Cooler ON_OFF.vi"("error in (no error)"=w10091, "Cooler ON/OFF"=w10083, "Interface in"=w10092) -> ("error out"=w10095:errorcluster, "Interface out"=w10097:refnum<class "Interface.lvclass">)  [unwired: 7 in]
            n4333 = call-dynamic "Write Interface.vi"("error in (no error)"=w10095, "Interface.lvclass"=w10097, "Channel in"=w10099) -> ("error out"=w10094:errorcluster, "Channel out"=w10098:refnum<class "Channel.lvclass">)  [unwired: 7 in]
            n4334 = call-dynamic "Read State Machine.vi"("error in (no error)"=w10094, "Device in"=w10098) -> ("error out"=w10110:errorcluster, "State Machine.lvclass"=w10111:refnum<class "State Machine.lvclass">, "Device out"=w10107:refnum<class "Channel.lvclass">)  [unwired: 7 in]
            n4335 = call "Next State.vi"("error in (no error)"=w10110, "New_State"=u32 30, "State Machine in"=w10111) -> ("error out"=w10105:errorcluster, "State Machine out"=w10108:refnum<class "State Machine.lvclass">)  [unwired: 7 in]
            n4336 = call-dynamic "Write State Machine.vi"("error in (no error)"=w10105, "State Machine.lvclass"=w10108, "Device in"=w10107) -> ("error out"=w10101:errorcluster, "Device out"=w10093:refnum<class "Channel.lvclass">)  [unwired: 7 in]
            n4337 = call-dynamic "Write Channel.vi"("error in (no error)"=w10101, "Channel.lvclass"=w10093, "Acquisition in"=w10106) -> ("error out"=w10102:errorcluster, "Acquisition out"=w10104:refnum<class "Acquisition.lvclass">)  [unwired: 7 in]
            n4338 = call "Write AcquisitionB.vi"("error in (no error)"=w10102, "Acquisition.lvclass"=w10104, "S4ACS_GUI in"=w10103) -> ("error out"=w10115:errorcluster, "S4ACS_GUI out"=w10114:refnum<class "S4GUI.lvclass">)  [unwired: 7 in]
          }
        }
      }
      event "cooler ON 3": Value Change {
        n4339 = event-data() -> ("NewVal"=w10116:bool)  [unwired: 1 in]
        n4340 = case shown="True" w10116 {
          tunnel: [w10121 w10156] -> w10120
          tunnel: [w10122 w10155] -> w10119
          tunnel: w10118 -> [w10122 w10126]
          tunnel: w10117 -> [w10121 w10125]
          frame False {
          }
          frame True {
            w10124 = i16 1 items=["Cooler OFF", "Cooler ON"] ("Cooler ON/OFF")
            n4341 = Concatenate Strings("SET COOLER " ("User Event"), "ON ", "CLICKED - CH3" ("User Event")) -> (w10128:string)
            n4342 = call-dynamic "Write User Event.vi"("error in (no error)"=w10125, "User Event"=w10128, "S4GUI in"=w10126) -> ("error out"=w10129:errorcluster, "S4GUI out"=w10131:refnum<class "S4GUI.lvclass">)  [unwired: 7 in]
            n4343 = call-dynamic "Read AcquisitionC.vi"("error in (no error)"=w10129, "S4ACS_GUI in"=w10131) -> ("error out"=w10153:errorcluster, "Acquisition.lvclass"=w10154:refnum<class "Acquisition.lvclass">, "S4ACS_GUI out"=w10144:refnum<class "S4GUI.lvclass">)  [unwired: 7 in]
            n4344 = call-dynamic "Read Channel.vi"("error in (no error)"=w10153, "Acquisition in"=w10154) -> ("error out"=w10137:errorcluster, "Channel.lvclass"=w10141:refnum<class "Channel.lvclass">, "Acquisition out"=w10147:refnum<class "Acquisition.lvclass">)  [unwired: 7 in]
            n4345 = call-dynamic "Read Interface.vi"("error in (no error)"=w10137, "Channel in"=w10141) -> ("error out"=w10132:errorcluster, "Interface.lvclass"=w10133:refnum<class "Interface.lvclass">, "Channel out"=w10140:refnum<class "Channel.lvclass">)  [unwired: 7 in]
            n4346 = call-dynamic "Write Cooler ON_OFF.vi"("error in (no error)"=w10132, "Cooler ON/OFF"=w10124, "Interface in"=w10133) -> ("error out"=w10136:errorcluster, "Interface out"=w10138:refnum<class "Interface.lvclass">)  [unwired: 7 in]
            n4347 = call-dynamic "Write Interface.vi"("error in (no error)"=w10136, "Interface.lvclass"=w10138, "Channel in"=w10140) -> ("error out"=w10135:errorcluster, "Channel out"=w10139:refnum<class "Channel.lvclass">)  [unwired: 7 in]
            n4348 = call-dynamic "Read State Machine.vi"("error in (no error)"=w10135, "Device in"=w10139) -> ("error out"=w10151:errorcluster, "State Machine.lvclass"=w10152:refnum<class "State Machine.lvclass">, "Device out"=w10148:refnum<class "Channel.lvclass">)  [unwired: 7 in]
            n4349 = call "Next State.vi"("error in (no error)"=w10151, "New_State"=u32 30, "State Machine in"=w10152) -> ("error out"=w10146:errorcluster, "State Machine out"=w10149:refnum<class "State Machine.lvclass">)  [unwired: 7 in]
            n4350 = call-dynamic "Write State Machine.vi"("error in (no error)"=w10146, "State Machine.lvclass"=w10149, "Device in"=w10148) -> ("error out"=w10142:errorcluster, "Device out"=w10134:refnum<class "Channel.lvclass">)  [unwired: 7 in]
            n4351 = call-dynamic "Write Channel.vi"("error in (no error)"=w10142, "Channel.lvclass"=w10134, "Acquisition in"=w10147) -> ("error out"=w10143:errorcluster, "Acquisition out"=w10145:refnum<class "Acquisition.lvclass">)  [unwired: 7 in]
            n4352 = call-dynamic "Write AcquisitionC.vi"("error in (no error)"=w10143, "Acquisition.lvclass"=w10145, "S4ACS_GUI in"=w10144) -> ("error out"=w10156:errorcluster, "S4ACS_GUI out"=w10155:refnum<class "S4GUI.lvclass">)  [unwired: 7 in]
          }
        }
      }
      event "cooler ON 4": Value Change {
        n4353 = event-data() -> ("NewVal"=w10157:bool)  [unwired: 1 in]
        n4354 = case shown="True" w10157 {
          tunnel: [w10162 w10197] -> w10161
          tunnel: [w10163 w10196] -> w10160
          tunnel: w10159 -> [w10163 w10167]
          tunnel: w10158 -> [w10162 w10166]
          frame False {
          }
          frame True {
            w10165 = i16 1 items=["Cooler OFF", "Cooler ON"] ("Cooler ON/OFF")
            n4355 = Concatenate Strings("SET COOLER " ("User Event"), "ON ", "CLICKED - CH4" ("User Event")) -> (w10169:string)
            n4356 = call-dynamic "Write User Event.vi"("error in (no error)"=w10166, "User Event"=w10169, "S4GUI in"=w10167) -> ("error out"=w10170:errorcluster, "S4GUI out"=w10172:refnum<class "S4GUI.lvclass">)  [unwired: 7 in]
            n4357 = call-dynamic "Read AcquisitionD.vi"("error in (no error)"=w10170, "S4ACS_GUI in"=w10172) -> ("error out"=w10194:errorcluster, "Acquisition.lvclass"=w10195:refnum<class "Acquisition.lvclass">, "S4ACS_GUI out"=w10185:refnum<class "S4GUI.lvclass">)  [unwired: 7 in]
            n4358 = call-dynamic "Read Channel.vi"("error in (no error)"=w10194, "Acquisition in"=w10195) -> ("error out"=w10178:errorcluster, "Channel.lvclass"=w10182:refnum<class "Channel.lvclass">, "Acquisition out"=w10188:refnum<class "Acquisition.lvclass">)  [unwired: 7 in]
            n4359 = call-dynamic "Read Interface.vi"("error in (no error)"=w10178, "Channel in"=w10182) -> ("error out"=w10173:errorcluster, "Interface.lvclass"=w10174:refnum<class "Interface.lvclass">, "Channel out"=w10181:refnum<class "Channel.lvclass">)  [unwired: 7 in]
            n4360 = call-dynamic "Write Cooler ON_OFF.vi"("error in (no error)"=w10173, "Cooler ON/OFF"=w10165, "Interface in"=w10174) -> ("error out"=w10177:errorcluster, "Interface out"=w10179:refnum<class "Interface.lvclass">)  [unwired: 7 in]
            n4361 = call-dynamic "Write Interface.vi"("error in (no error)"=w10177, "Interface.lvclass"=w10179, "Channel in"=w10181) -> ("error out"=w10176:errorcluster, "Channel out"=w10180:refnum<class "Channel.lvclass">)  [unwired: 7 in]
            n4362 = call-dynamic "Read State Machine.vi"("error in (no error)"=w10176, "Device in"=w10180) -> ("error out"=w10192:errorcluster, "State Machine.lvclass"=w10193:refnum<class "State Machine.lvclass">, "Device out"=w10189:refnum<class "Channel.lvclass">)  [unwired: 7 in]
            n4363 = call "Next State.vi"("error in (no error)"=w10192, "New_State"=u32 30, "State Machine in"=w10193) -> ("error out"=w10187:errorcluster, "State Machine out"=w10190:refnum<class "State Machine.lvclass">)  [unwired: 7 in]
            n4364 = call-dynamic "Write State Machine.vi"("error in (no error)"=w10187, "State Machine.lvclass"=w10190, "Device in"=w10189) -> ("error out"=w10183:errorcluster, "Device out"=w10175:refnum<class "Channel.lvclass">)  [unwired: 7 in]
            n4365 = call-dynamic "Write Channel.vi"("error in (no error)"=w10183, "Channel.lvclass"=w10175, "Acquisition in"=w10188) -> ("error out"=w10184:errorcluster, "Acquisition out"=w10186:refnum<class "Acquisition.lvclass">)  [unwired: 7 in]
            n4366 = call-dynamic "Write AcquisitionD.vi"("error in (no error)"=w10184, "Acquisition.lvclass"=w10186, "S4ACS_GUI in"=w10185) -> ("error out"=w10197:errorcluster, "S4ACS_GUI out"=w10196:refnum<class "S4GUI.lvclass">)  [unwired: 7 in]
          }
        }
      }
      event "cooler OFF 1": Value Change {
        n4367 = event-data() -> ("NewVal"=w10198:bool)  [unwired: 1 in]
        n4368 = case shown="True" w10198 {
          tunnel: [w10203 w10238] -> w10202
          tunnel: [w10204 w10237] -> w10201
          tunnel: w10200 -> [w10204 w10208]
          tunnel: w10199 -> [w10203 w10207]
          frame False {
          }
          frame True {
            w10206 = i16 0 items=["Cooler OFF", "Cooler ON"] ("Cooler ON/OFF")
            n4369 = Concatenate Strings("SET COOLER " ("User Event"), "OFF ", "CLICKED - CH1" ("User Event")) -> (w10210:string)
            n4370 = call-dynamic "Write User Event.vi"("error in (no error)"=w10207, "User Event"=w10210, "S4GUI in"=w10208) -> ("error out"=w10211:errorcluster, "S4GUI out"=w10213:refnum<class "S4GUI.lvclass">)  [unwired: 7 in]
            n4371 = call-dynamic "Read AcquisitionA.vi"("error in (no error)"=w10211, "S4ACS_GUI in"=w10213) -> ("error out"=w10235:errorcluster, "Acquisition.lvclass"=w10236:refnum<class "Acquisition.lvclass">, "S4ACS_GUI out"=w10226:refnum<class "S4GUI.lvclass">)  [unwired: 7 in]
            n4372 = call-dynamic "Read Channel.vi"("error in (no error)"=w10235, "Acquisition in"=w10236) -> ("error out"=w10219:errorcluster, "Channel.lvclass"=w10223:refnum<class "Channel.lvclass">, "Acquisition out"=w10229:refnum<class "Acquisition.lvclass">)  [unwired: 7 in]
            n4373 = call-dynamic "Read Interface.vi"("error in (no error)"=w10219, "Channel in"=w10223) -> ("error out"=w10214:errorcluster, "Interface.lvclass"=w10215:refnum<class "Interface.lvclass">, "Channel out"=w10222:refnum<class "Channel.lvclass">)  [unwired: 7 in]
            n4374 = call-dynamic "Write Cooler ON_OFF.vi"("error in (no error)"=w10214, "Cooler ON/OFF"=w10206, "Interface in"=w10215) -> ("error out"=w10218:errorcluster, "Interface out"=w10220:refnum<class "Interface.lvclass">)  [unwired: 7 in]
            n4375 = call-dynamic "Write Interface.vi"("error in (no error)"=w10218, "Interface.lvclass"=w10220, "Channel in"=w10222) -> ("error out"=w10217:errorcluster, "Channel out"=w10221:refnum<class "Channel.lvclass">)  [unwired: 7 in]
            n4376 = call-dynamic "Read State Machine.vi"("error in (no error)"=w10217, "Device in"=w10221) -> ("error out"=w10233:errorcluster, "State Machine.lvclass"=w10234:refnum<class "State Machine.lvclass">, "Device out"=w10230:refnum<class "Channel.lvclass">)  [unwired: 7 in]
            n4377 = call "Next State.vi"("error in (no error)"=w10233, "New_State"=u32 30, "State Machine in"=w10234) -> ("error out"=w10228:errorcluster, "State Machine out"=w10231:refnum<class "State Machine.lvclass">)  [unwired: 7 in]
            n4378 = call-dynamic "Write State Machine.vi"("error in (no error)"=w10228, "State Machine.lvclass"=w10231, "Device in"=w10230) -> ("error out"=w10224:errorcluster, "Device out"=w10216:refnum<class "Channel.lvclass">)  [unwired: 7 in]
            n4379 = call-dynamic "Write Channel.vi"("error in (no error)"=w10224, "Channel.lvclass"=w10216, "Acquisition in"=w10229) -> ("error out"=w10225:errorcluster, "Acquisition out"=w10227:refnum<class "Acquisition.lvclass">)  [unwired: 7 in]
            n4380 = call-dynamic "Write AcquisitionA.vi"("error in (no error)"=w10225, "Acquisition.lvclass"=w10227, "S4ACS_GUI in"=w10226) -> ("error out"=w10238:errorcluster, "S4ACS_GUI out"=w10237:refnum<class "S4GUI.lvclass">)  [unwired: 7 in]
          }
        }
      }
      event "cooler OFF 2": Value Change {
        n4381 = event-data() -> ("NewVal"=w10239:bool)  [unwired: 1 in]
        n4382 = case shown="True" w10239 {
          tunnel: [w10244 w10279] -> w10243
          tunnel: [w10245 w10278] -> w10242
          tunnel: w10241 -> [w10245 w10249]
          tunnel: w10240 -> [w10244 w10248]
          frame False {
          }
          frame True {
            w10247 = i16 0 items=["Cooler OFF", "Cooler ON"] ("Cooler ON/OFF")
            n4383 = Concatenate Strings("SET COOLER " ("User Event"), "OFF ", "CLICKED - CH2" ("User Event")) -> (w10251:string)
            n4384 = call-dynamic "Write User Event.vi"("error in (no error)"=w10248, "User Event"=w10251, "S4GUI in"=w10249) -> ("error out"=w10252:errorcluster, "S4GUI out"=w10254:refnum<class "S4GUI.lvclass">)  [unwired: 7 in]
            n4385 = call "Read AcquisitionB.vi"("error in (no error)"=w10252, "S4ACS_GUI in"=w10254) -> ("error out"=w10276:errorcluster, "Acquisition.lvclass"=w10277:refnum<class "Acquisition.lvclass">, "S4ACS_GUI out"=w10267:refnum<class "S4GUI.lvclass">)  [unwired: 7 in]
            n4386 = call-dynamic "Read Channel.vi"("error in (no error)"=w10276, "Acquisition in"=w10277) -> ("error out"=w10260:errorcluster, "Channel.lvclass"=w10264:refnum<class "Channel.lvclass">, "Acquisition out"=w10270:refnum<class "Acquisition.lvclass">)  [unwired: 7 in]
            n4387 = call-dynamic "Read Interface.vi"("error in (no error)"=w10260, "Channel in"=w10264) -> ("error out"=w10255:errorcluster, "Interface.lvclass"=w10256:refnum<class "Interface.lvclass">, "Channel out"=w10263:refnum<class "Channel.lvclass">)  [unwired: 7 in]
            n4388 = call-dynamic "Write Cooler ON_OFF.vi"("error in (no error)"=w10255, "Cooler ON/OFF"=w10247, "Interface in"=w10256) -> ("error out"=w10259:errorcluster, "Interface out"=w10261:refnum<class "Interface.lvclass">)  [unwired: 7 in]
            n4389 = call-dynamic "Write Interface.vi"("error in (no error)"=w10259, "Interface.lvclass"=w10261, "Channel in"=w10263) -> ("error out"=w10258:errorcluster, "Channel out"=w10262:refnum<class "Channel.lvclass">)  [unwired: 7 in]
            n4390 = call-dynamic "Read State Machine.vi"("error in (no error)"=w10258, "Device in"=w10262) -> ("error out"=w10274:errorcluster, "State Machine.lvclass"=w10275:refnum<class "State Machine.lvclass">, "Device out"=w10271:refnum<class "Channel.lvclass">)  [unwired: 7 in]
            n4391 = call "Next State.vi"("error in (no error)"=w10274, "New_State"=u32 30, "State Machine in"=w10275) -> ("error out"=w10269:errorcluster, "State Machine out"=w10272:refnum<class "State Machine.lvclass">)  [unwired: 7 in]
            n4392 = call-dynamic "Write State Machine.vi"("error in (no error)"=w10269, "State Machine.lvclass"=w10272, "Device in"=w10271) -> ("error out"=w10265:errorcluster, "Device out"=w10257:refnum<class "Channel.lvclass">)  [unwired: 7 in]
            n4393 = call-dynamic "Write Channel.vi"("error in (no error)"=w10265, "Channel.lvclass"=w10257, "Acquisition in"=w10270) -> ("error out"=w10266:errorcluster, "Acquisition out"=w10268:refnum<class "Acquisition.lvclass">)  [unwired: 7 in]
            n4394 = call "Write AcquisitionB.vi"("error in (no error)"=w10266, "Acquisition.lvclass"=w10268, "S4ACS_GUI in"=w10267) -> ("error out"=w10279:errorcluster, "S4ACS_GUI out"=w10278:refnum<class "S4GUI.lvclass">)  [unwired: 7 in]
          }
        }
      }
      event "cooler OFF 3": Value Change {
        n4395 = event-data() -> ("NewVal"=w10280:bool)  [unwired: 1 in]
        n4396 = case shown="True" w10280 {
          tunnel: [w10285 w10320] -> w10284
          tunnel: [w10286 w10319] -> w10283
          tunnel: w10282 -> [w10286 w10290]
          tunnel: w10281 -> [w10285 w10289]
          frame False {
          }
          frame True {
            w10288 = i16 0 items=["Cooler OFF", "Cooler ON"] ("Cooler ON/OFF")
            n4397 = Concatenate Strings("SET COOLER " ("User Event"), "OFF ", "CLICKED - CH3" ("User Event")) -> (w10292:string)
            n4398 = call-dynamic "Write User Event.vi"("error in (no error)"=w10289, "User Event"=w10292, "S4GUI in"=w10290) -> ("error out"=w10293:errorcluster, "S4GUI out"=w10295:refnum<class "S4GUI.lvclass">)  [unwired: 7 in]
            n4399 = call-dynamic "Read AcquisitionC.vi"("error in (no error)"=w10293, "S4ACS_GUI in"=w10295) -> ("error out"=w10317:errorcluster, "Acquisition.lvclass"=w10318:refnum<class "Acquisition.lvclass">, "S4ACS_GUI out"=w10308:refnum<class "S4GUI.lvclass">)  [unwired: 7 in]
            n4400 = call-dynamic "Read Channel.vi"("error in (no error)"=w10317, "Acquisition in"=w10318) -> ("error out"=w10301:errorcluster, "Channel.lvclass"=w10305:refnum<class "Channel.lvclass">, "Acquisition out"=w10311:refnum<class "Acquisition.lvclass">)  [unwired: 7 in]
            n4401 = call-dynamic "Read Interface.vi"("error in (no error)"=w10301, "Channel in"=w10305) -> ("error out"=w10296:errorcluster, "Interface.lvclass"=w10297:refnum<class "Interface.lvclass">, "Channel out"=w10304:refnum<class "Channel.lvclass">)  [unwired: 7 in]
            n4402 = call-dynamic "Write Cooler ON_OFF.vi"("error in (no error)"=w10296, "Cooler ON/OFF"=w10288, "Interface in"=w10297) -> ("error out"=w10300:errorcluster, "Interface out"=w10302:refnum<class "Interface.lvclass">)  [unwired: 7 in]
            n4403 = call-dynamic "Write Interface.vi"("error in (no error)"=w10300, "Interface.lvclass"=w10302, "Channel in"=w10304) -> ("error out"=w10299:errorcluster, "Channel out"=w10303:refnum<class "Channel.lvclass">)  [unwired: 7 in]
            n4404 = call-dynamic "Read State Machine.vi"("error in (no error)"=w10299, "Device in"=w10303) -> ("error out"=w10315:errorcluster, "State Machine.lvclass"=w10316:refnum<class "State Machine.lvclass">, "Device out"=w10312:refnum<class "Channel.lvclass">)  [unwired: 7 in]
            n4405 = call "Next State.vi"("error in (no error)"=w10315, "New_State"=u32 30, "State Machine in"=w10316) -> ("error out"=w10310:errorcluster, "State Machine out"=w10313:refnum<class "State Machine.lvclass">)  [unwired: 7 in]
            n4406 = call-dynamic "Write State Machine.vi"("error in (no error)"=w10310, "State Machine.lvclass"=w10313, "Device in"=w10312) -> ("error out"=w10306:errorcluster, "Device out"=w10298:refnum<class "Channel.lvclass">)  [unwired: 7 in]
            n4407 = call-dynamic "Write Channel.vi"("error in (no error)"=w10306, "Channel.lvclass"=w10298, "Acquisition in"=w10311) -> ("error out"=w10307:errorcluster, "Acquisition out"=w10309:refnum<class "Acquisition.lvclass">)  [unwired: 7 in]
            n4408 = call-dynamic "Write AcquisitionC.vi"("error in (no error)"=w10307, "Acquisition.lvclass"=w10309, "S4ACS_GUI in"=w10308) -> ("error out"=w10320:errorcluster, "S4ACS_GUI out"=w10319:refnum<class "S4GUI.lvclass">)  [unwired: 7 in]
          }
        }
      }
      event "cooler OFF 4": Value Change {
        n4409 = event-data() -> ("NewVal"=w10321:bool)  [unwired: 1 in]
        n4410 = case shown="True" w10321 {
          tunnel: [w10326 w10361] -> w10325
          tunnel: [w10327 w10360] -> w10324
          tunnel: w10323 -> [w10327 w10331]
          tunnel: w10322 -> [w10326 w10330]
          frame False {
          }
          frame True {
            w10329 = i16 0 items=["Cooler OFF", "Cooler ON"] ("Cooler ON/OFF")
            n4411 = Concatenate Strings("SET COOLER " ("User Event"), "OFF ", "CLICKED - CH4" ("User Event")) -> (w10333:string)
            n4412 = call-dynamic "Write User Event.vi"("error in (no error)"=w10330, "User Event"=w10333, "S4GUI in"=w10331) -> ("error out"=w10334:errorcluster, "S4GUI out"=w10336:refnum<class "S4GUI.lvclass">)  [unwired: 7 in]
            n4413 = call-dynamic "Read AcquisitionD.vi"("error in (no error)"=w10334, "S4ACS_GUI in"=w10336) -> ("error out"=w10358:errorcluster, "Acquisition.lvclass"=w10359:refnum<class "Acquisition.lvclass">, "S4ACS_GUI out"=w10349:refnum<class "S4GUI.lvclass">)  [unwired: 7 in]
